vi "Read Bit Array.vi"(11 "GDSII.DataType.Bit Array in":refnum<class "GDSII.DataType.Bit Array.lvclass">) -> (2 "Bit Array":i16[](array[numeric]), 3 "GDSII.DataType.Bit Array out":refnum<class "GDSII.DataType.Bit Array.lvclass">)   [LabVIEW 2019, in "GDSII.DataType.Bit Array.lvclass"]
uses:
  GDSII.DataType.Bit Array.lvclass
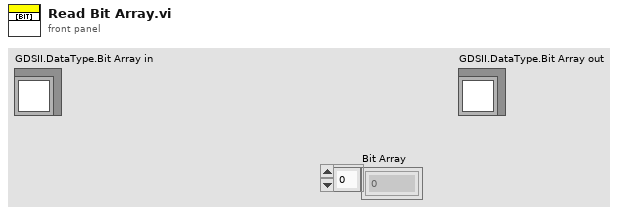
[diagram p1: front panel]
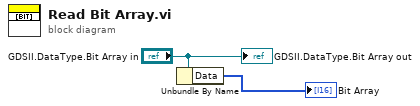
[diagram p0: block diagram]
diagram:
  n1 = Unbundle By Name("GDSII.DataType.Bit Array in") -> ("Data"=→"Bit Array":i16[])
  "GDSII.DataType.Bit Array out" <- "GDSII.DataType.Bit Array in"
